vi "twomotor_v2.vi"() -> ()   [LabVIEW 2014]
uses:
  <vilib>/rvi/FXPMathLib/FxpSinAndCos/subVIs/nifxpmath_SinAndCos_SimConfig.ctl
  <vilib>/rvi/Emulation/niFpgaGetClockAttributes.vi
  <vilib>/rvi/Emulation/niFpgaSctlEmulationGetInTimedLoop.vi
  <vilib>/rvi/Emulation/niFpgaEmulationReportErrorSimple.vi
  <vilib>/rvi/eio/common/nirviEmuTemplateMethod_errors.vi
  <vilib>/rvi/Emulation/niFpgaProcessEmulError.vi
  <vilib>/rvi/Emulation/niFpgaCriticalErrorInLSC.vi
  <vilib>/rvi/FXPMathLib/FxpSinAndCos/simVIs/DllFxpSinAndCosTemp_sub.vi
  <vilib>/eio/EIONode/EIONode.xnode
  <vilib>/rvi/FXPMathLib/FxpMul/XNode/nifxpmath_Multiplier.xnode
  <vilib>/rvi/FXPMathLib/FxpSinAndCos/XNode/nifxpmath_SinAndCos.xnode
  <vilib>/rvi/FXPMathLib/sim/FxpSim.dll
panel:
  in  "Direction_y":bool
  in  "Direction_p":bool
  out "va_y":fxp<+/-,37,8>
  out "vb_y":fxp<+/-,37,8>
  in  "stop motor_y":bool
  out "vq_y":fxp<+/-,20,5> format="%.57g"
  out "vd_y":fxp<+/-,20,5>
  in  "Fmr_y":fxp<+/-,21,11>
  out "Dp_d (mm/s)":fxp<+/-,46,10>
  out "omega_p (rad/s)":fxp<+/-,20,9>
  out "mt_y":u32
  in  "mt0_y":u32
  in  "Encoder Reset_y":bool
  out "rad_y(NrTheta)":fxp<+/-,32,2>
  out "D_y(mm)":fxp<+/-,32,2>
  out "Encoder Position_y":i32
  in  "Ini coe.":bool
  out "va_p":fxp<+/-,38,8>
  out "vb_p":fxp<+/-,38,8>
  in  "stop motor_p":bool
  in  "Fmr_p":fxp<+/-,21,11>
  out "vq_p":fxp<+/-,20,5> format="%.57g"
  out "vd_p":fxp<+/-,20,5>
  out "Dy_d (mm/s)":fxp<+/-,32,12>
  out "mt_p":u32
  out "omega_y (rad/s)":fxp<+/-,32,18>
  in  "mt0_p":u32
  out "D_p(mm)":fxp<+/-,22,7>
  out "rad_p(NrTheta)":fxp<+/-,33,18>
  out "Encoder Position_p":i32
  in  "Encoder Reset_p":bool
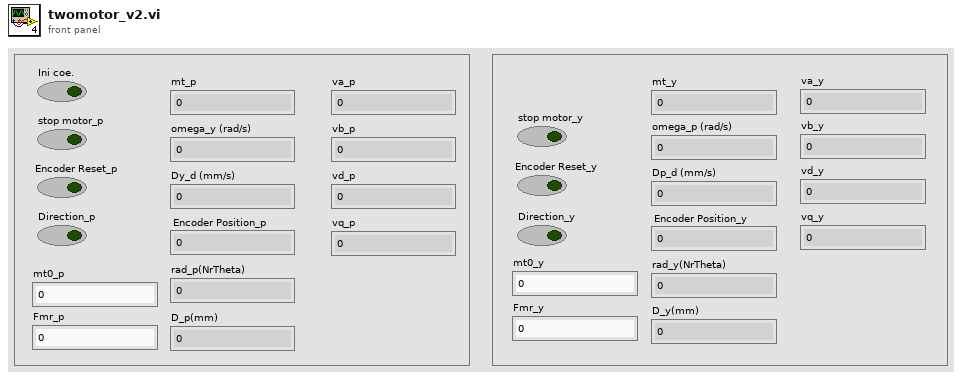
[diagram p1: front panel]
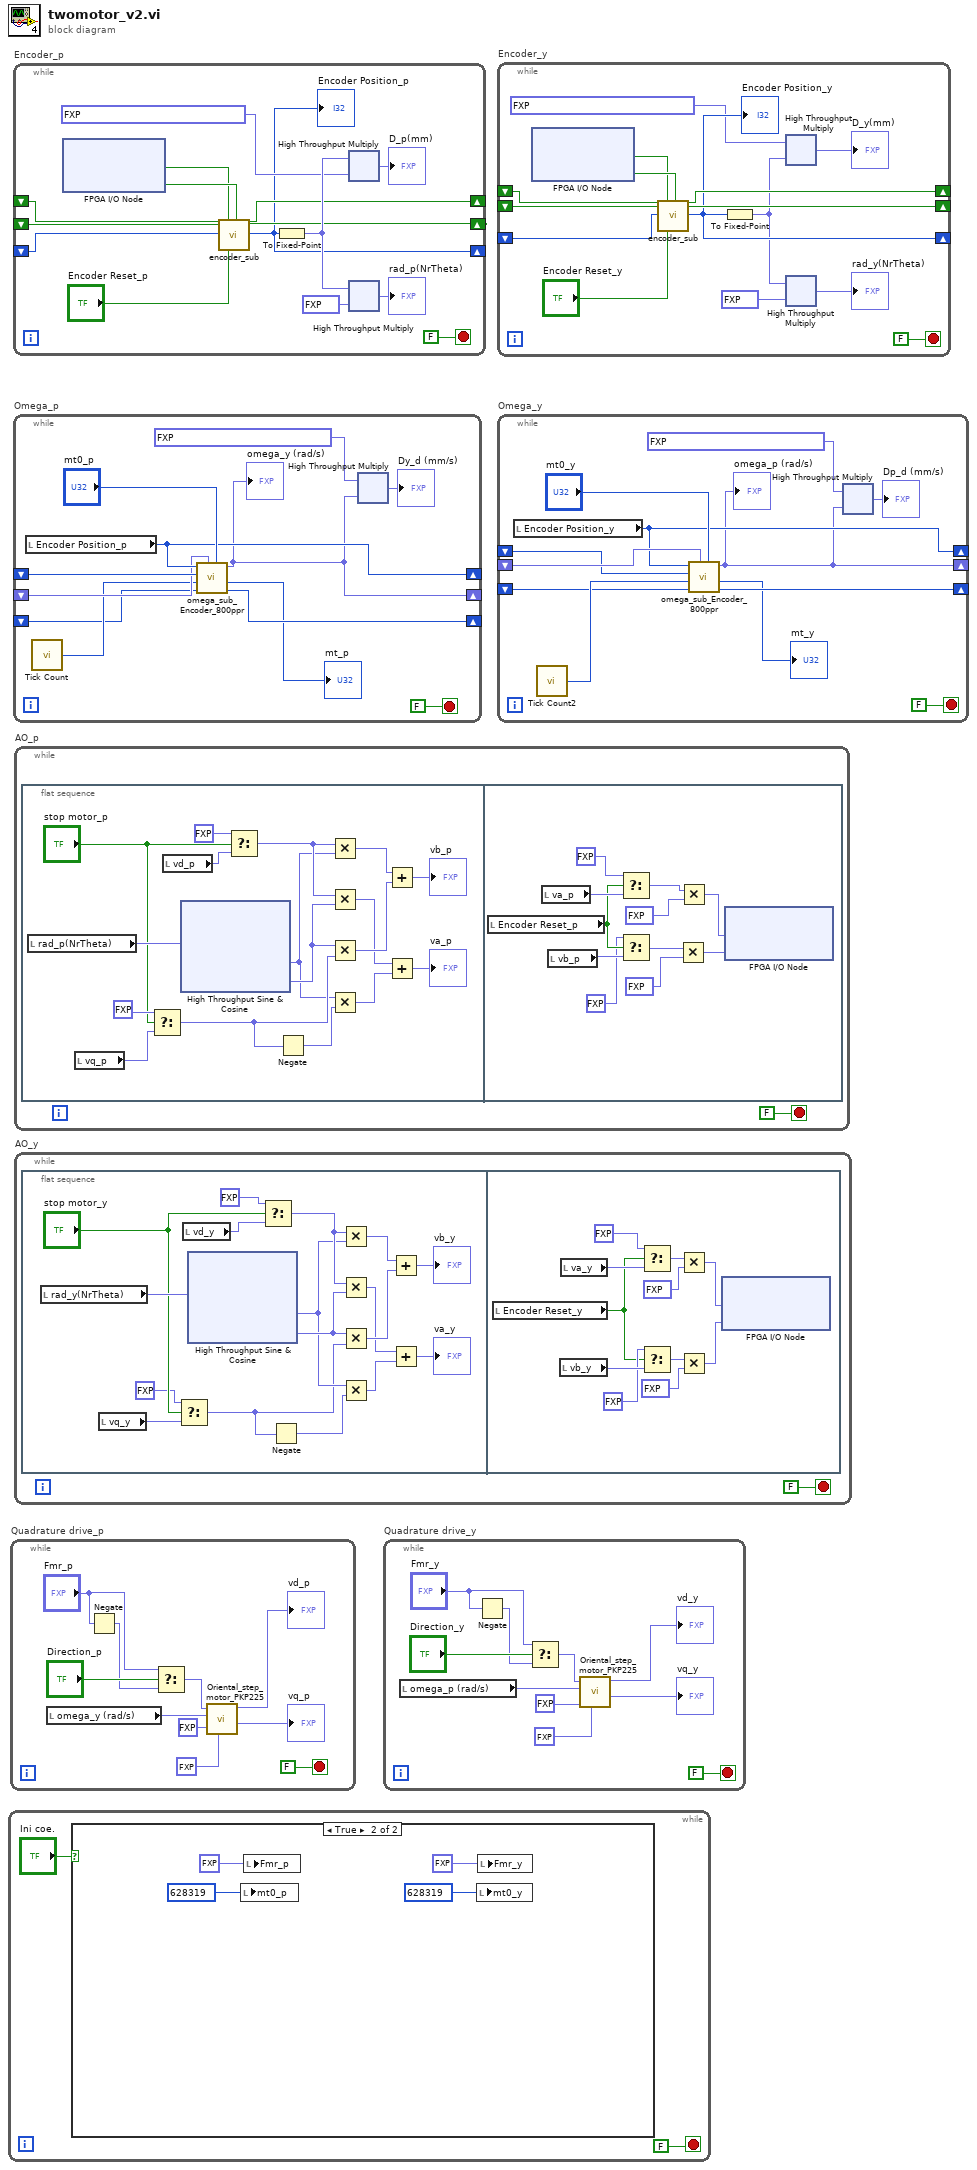
[diagram p0: block diagram]
diagram:
  n1 = while {
    stop <- FALSE stop-if-true
    n2 = case shown="True" "Ini coe." {
      frame False {
      }
      frame True {
        n3 = local write "mt0_p"(u32 628319 ("mt0")) -> ()
        n4 = local write "Fmr_p"(fxp<+/-,21,11> 50.0 ("Fmr")) -> ()
        n5 = local write "mt0_y"(u32 628319 ("mt0")) -> ()
        n6 = local write "Fmr_y"(fxp<+/-,21,11> 50.0 ("Fmr")) -> ()
      }
    }
  }
  n7 = while "Quadrature drive_p" {
    stop <- FALSE stop-if-true
    n8 = local read "omega_y (rad/s)"() -> (w12:fxp<+/-,32,18>)
    n9 = Negate(x="Fmr_p") -> (-x=w7:fxp<+/-,22,12>)
    n10 = Select(t="Fmr_p", s="Direction_p", f=w7) -> (s? t:f=w10:fxp<+/-,22,12>)
    n11 = call "Oriental_step_motor_PKP225.vi"("F_Threshold"=fxp<+,12,12> 10.0, "dFmr"=fxp<+/-,25,15> 0.0, "omega"=w12, "Fmr"=w10) -> ("vq_F"=→"vq_p":fxp<+/-,20,5>, "vd_F"=→"vd_p":fxp<+/-,20,5>)  [unwired: 6 in]
  }
  n12 = while "Encoder_p" {
    shift-right: [w23] -> _
    shift-left: _ -> [w25]
    shift-right: [w22] -> _
    shift-left: _ -> [w24]
    shift-right: [w20] -> _
    shift-left: _ -> [w21]
    stop <- FALSE stop-if-true
    n13 = xnode "FPGA I/O Node"() -> ("Mod4/DI3"=w30:bool, "Mod4/DI4"=w31:bool)  [unwired: 2 in, 2 out]
    n14 = call "encoder_sub.vi"("A_pre"=w25, "B_pre"=w24, "Encoder Position_pre"=w21, "A input"=w30, "Encoder Position Reset"="Encoder Reset_p", "B input"=w31) -> ("A"=w23:bool, "B"=w22:bool, "Encoder Position (Counts)"=w20:i32)  [unwired: 19 in]
    "Encoder Position_p" <- w20
    n15 = To Fixed-Point(number=w20) -> (fixed-point=w28:fxp<+/-,32,32>)  [unwired: 1 in]
    n16 = xnode ("High Throughput Multiply")("x"=w28, "y"=fxp<+/-,24,0> 0.002499997615814209) -> ("x*y"=→"D_p(mm)":fxp<+/-,56,32>)
    n17 = xnode ("High Throughput Multiply")("x"=w28, "y"=fxp<+/-,24,0> 0.125) -> ("x*y"=→"rad_p(NrTheta)":fxp<+/-,56,32>)
  }
  n18 = while "Omega_p" {
    shift-right: [w41] -> _
    shift-left: _ -> [w42]
    shift-right: [w34] -> _
    shift-left: _ -> [w40]
    shift-right: [w37] -> _
    shift-left: _ -> [w38]
    stop <- FALSE stop-if-true
    n19 = local read "Encoder Position_p"() -> (w41:i32)
    n20 = call "Tick Count"() -> ("Tick Count(Ticks)"=w39:u32)
    n21 = call "omega_sub_Encoder_800ppr.vi"("mt0"="mt0_p", "omega_pre"=w40, "ticks_m_pre"=w38, "ticks"=w39, "count_pre"=w42, "count"=w41) -> ("ticks_m"=w37:u32, "mt"=→"mt_p":u32, "omega"=w34:fxp<+/-,20,9>)  [unwired: 3 in]
    "omega_y (rad/s)" <- w34
    n22 = xnode ("High Throughput Multiply")("x"=fxp<+/-,26,1> 0.3183099031448364, "y"=w34) -> ("x*y"=→"Dy_d (mm/s)":fxp<+/-,46,10>)
  }
  n23 = while "AO_p" {
    stop <- FALSE stop-if-true
    n24 = flat-sequence {
      frame #0 {
        n25 = local read "rad_p(NrTheta)"() -> (w60:fxp<+/-,33,18>)
        n26 = local read "vq_p"() -> (w58:fxp<+/-,20,5>)
        n27 = Select(t=fxp<+,20,5> 0.0, s="stop motor_p", f=w58) -> (s? t:f=w55:fxp<+/-,21,6>)
        n28 = local read "vd_p"() -> (w59:fxp<+/-,20,5>)
        n29 = xnode "High Throughput Sine & Cosine"("x (pi)"=w60) -> ("sin(x)"=w51:fxp<+/-,17,2>, "cos(x)"=w53:fxp<+/-,17,2>)
        n30 = Select(t=fxp<+,20,5> 0.0, s="stop motor_p", f=w59) -> (s? t:f=w52:fxp<+/-,21,6>)
        n31 = Negate(x=w55) -> (-x=w54:fxp<+/-,21,6>)
        n32 = Multiply(x=w52, y=w51) -> (x*y=w50:fxp<+/-,37,7>)
        n33 = Multiply(x=w52, y=w53) -> (x*y=w48:fxp<+/-,37,7>)
        n34 = Multiply(x=w53, y=w55) -> (x*y=w49:fxp<+/-,37,7>)
        n35 = Multiply(x=w51, y=w54) -> (x*y=w47:fxp<+/-,37,7>)
        n36 = Add(x=w50, y=w49) -> (x+y=→"vb_p":fxp<+/-,38,8>)
        n37 = Add(x=w48, y=w47) -> (x+y=→"va_p":fxp<+/-,38,8>)
      }
      frame #1 {
        n38 = local read "Encoder Reset_p"() -> (w94:bool)
        n39 = local read "va_p"() -> (w96:fxp<+/-,38,8>)
        n40 = local read "vb_p"() -> (w95:fxp<+/-,38,8>)
        n41 = Select(t=fxp<+/-,20,5> 5.0 ("y"), s=w94, f=w96) -> (s? t:f=w97:fxp<+/-,38,8>)
        n42 = Select(t=fxp<+/-,20,5> 0.0 ("y"), s=w94, f=w95) -> (s? t:f=w98:fxp<+/-,38,8>)
        n43 = Multiply(x=w98, y=fxp<+/-,20,5> -0.5) -> (x*y=w102:fxp<+/-,57,12>)
        n44 = Multiply(x=w97, y=fxp<+/-,20,5> -0.5) -> (x*y=w101:fxp<+/-,57,12>)
        n45 = xnode "FPGA I/O Node"("Mod8/AO0"=w101, "Mod8/AO1"=w102) -> ()  [unwired: 2 in, 2 out]
      }
    }
  }
  n46 = while "AO_y" {
    stop <- FALSE stop-if-true
    n47 = flat-sequence {
      frame #0 {
        n48 = local read "rad_y(NrTheta)"() -> (w120:fxp<+/-,32,2>)
        n49 = local read "vq_y"() -> (w110:fxp<+/-,20,5>)
        n50 = Select(t=fxp<+,20,5> 0.0, s="stop motor_y", f=w110) -> (s? t:f=w111:fxp<+/-,21,6>)
        n51 = local read "vd_y"() -> (w109:fxp<+/-,20,5>)
        n52 = xnode "High Throughput Sine & Cosine"("x (pi)"=w120) -> ("sin(x)"=w113:fxp<+/-,16,2>, "cos(x)"=w114:fxp<+/-,16,2>)
        n53 = Select(t=fxp<+,20,5> 0.0, s="stop motor_y", f=w109) -> (s? t:f=w115:fxp<+/-,21,6>)
        n54 = Negate(x=w111) -> (-x=w112:fxp<+/-,21,6>)
        n55 = Multiply(x=w115, y=w113) -> (x*y=w119:fxp<+/-,36,7>)
        n56 = Multiply(x=w115, y=w114) -> (x*y=w117:fxp<+/-,36,7>)
        n57 = Multiply(x=w114, y=w111) -> (x*y=w118:fxp<+/-,36,7>)
        n58 = Multiply(x=w113, y=w112) -> (x*y=w116:fxp<+/-,36,7>)
        n59 = Add(x=w119, y=w118) -> (x+y=→"vb_y":fxp<+/-,37,8>)
        n60 = Add(x=w117, y=w116) -> (x+y=→"va_y":fxp<+/-,37,8>)
      }
      frame #1 {
        n61 = local read "Encoder Reset_y"() -> (w153:bool)
        n62 = local read "vb_y"() -> (w160:fxp<+/-,37,8>)
        n63 = local read "va_y"() -> (w161:fxp<+/-,37,8>)
        n64 = Select(t=fxp<+/-,20,5> 5.0 ("y"), s=w153, f=w161) -> (s? t:f=w157:fxp<+/-,37,8>)
        n65 = Select(t=fxp<+/-,20,5> 0.0 ("y"), s=w153, f=w160) -> (s? t:f=w156:fxp<+/-,37,8>)
        n66 = Multiply(x=w157, y=fxp<+/-,20,5> -0.5) -> (x*y=w152:fxp<+/-,56,12>)
        n67 = Multiply(x=w156, y=fxp<+/-,20,5> -0.5) -> (x*y=w151:fxp<+/-,56,12>)
        n68 = xnode "FPGA I/O Node"("Mod8/AO2"=w152, "Mod8/AO3"=w151) -> ()  [unwired: 2 in, 2 out]
      }
    }
  }
  n69 = while "Quadrature drive_y" {
    stop <- FALSE stop-if-true
    n70 = local read "omega_p (rad/s)"() -> (w167:fxp<+/-,20,9>)
    n71 = Negate(x="Fmr_y") -> (-x=w164:fxp<+/-,22,12>)
    n72 = Select(t="Fmr_y", s="Direction_y", f=w164) -> (s? t:f=w163:fxp<+/-,22,12>)
    n73 = call "Oriental_step_motor_PKP225.vi"("F_Threshold"=fxp<+,12,12> 10.0, "dFmr"=fxp<+/-,25,15> 0.0, "omega"=w167, "Fmr"=w163) -> ("vq_F"=→"vq_y":fxp<+/-,20,5>, "vd_F"=→"vd_y":fxp<+/-,20,5>)  [unwired: 6 in]
  }
  n74 = while "Encoder_y" {
    shift-right: [w182] -> _
    shift-left: _ -> [w184]
    shift-right: [w181] -> _
    shift-left: _ -> [w183]
    shift-right: [w179] -> _
    shift-left: _ -> [w180]
    stop <- FALSE stop-if-true
    n75 = xnode "FPGA I/O Node"() -> ("Mod4/DI0"=w185:bool, "Mod4/DI1"=w186:bool)  [unwired: 2 in, 2 out]
    n76 = call "encoder_sub.vi"("A_pre"=w184, "B_pre"=w183, "Encoder Position_pre"=w180, "A input"=w185, "Encoder Position Reset"="Encoder Reset_y", "B input"=w186) -> ("A"=w182:bool, "B"=w181:bool, "Encoder Position (Counts)"=w179:i32)  [unwired: 19 in]
    "Encoder Position_y" <- w179
    n77 = To Fixed-Point(number=w179) -> (fixed-point=w174:fxp<+/-,32,32>)  [unwired: 1 in]
    n78 = xnode ("High Throughput Multiply")("x"=fxp<+/-,24,0> 0.002499997615814209 ("y"), "y"=w174) -> ("x*y"=→"D_y(mm)":fxp<+/-,56,32>)
    n79 = xnode ("High Throughput Multiply")("x"=w174, "y"=fxp<+/-,24,0> 0.125) -> ("x*y"=→"rad_y(NrTheta)":fxp<+/-,56,32>)
  }
  n80 = while "Omega_y" {
    shift-right: [w191] -> _
    shift-left: _ -> [w192]
    shift-right: [w189] -> _
    shift-left: _ -> [w197]
    shift-right: [w194] -> _
    shift-left: _ -> [w195]
    stop <- FALSE stop-if-true
    n81 = local read "Encoder Position_y"() -> (w191:i32)
    n82 = call "Tick Count2"() -> ("Tick Count(Ticks)"=w196:u32)
    n83 = call "omega_sub_Encoder_800ppr.vi"("mt0"="mt0_y", "omega_pre"=w197, "ticks_m_pre"=w195, "ticks"=w196, "count_pre"=w192, "count"=w191) -> ("ticks_m"=w194:u32, "mt"=→"mt_y":u32, "omega"=w189:fxp<+/-,20,9>)  [unwired: 3 in]
    "omega_p (rad/s)" <- w189
    n84 = xnode ("High Throughput Multiply")("x"=fxp<+/-,26,1> 0.3183099031448364, "y"=w189) -> ("x*y"=→"Dp_d (mm/s)":fxp<+/-,46,10>)
  }
